vi "Timeout Timer.vi"(2 "timeout(s)":dbl=5.0) -> (7 "timeout?":bool, 9 "time esliped?":dbl)   [LabVIEW 2017]
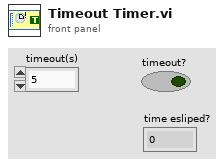
[diagram p1: front panel]
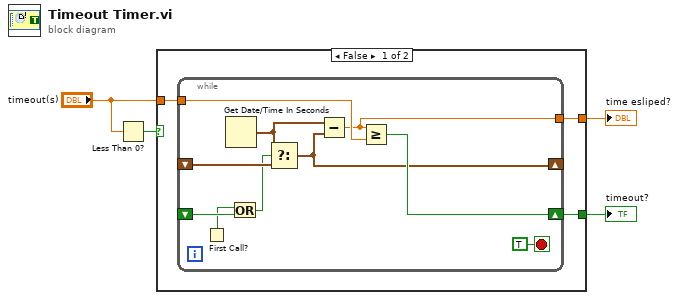
[diagram p0: block diagram]
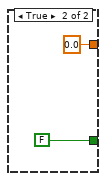
[diagram p2: hidden frame]
diagram:
  n1 = Less Than 0?(x="timeout(s)") -> (x < 0?=w3:bool)
  n2 = case shown="False" w3 {
    tunnel: "timeout(s)" -> [w7 _]
    tunnel: [w6 FALSE] -> w4
    tunnel: [w5 0.0] -> w1
    frame False {
      n3 = while {
        shift-right: [w8] -> _
        shift-left: _ -> [w16]
        tunnel: w7 -> [w15]
        shift-right: [w14] -> w6
        shift-left: _ -> [w13]
        tunnel: [w10] -> w5
        stop <- TRUE stop-if-true
        n4 = First Call?() -> (First Call?: T/F=w12:bool)
        n5 = Get Date/Time In Seconds() -> (seconds since 1Jan1904=w9:timestamp)
        n6 = Or(x=w12, y=w13) -> (x .or. y?=w11:bool)
        n7 = Select(t=w9, s=w11, f=w16) -> (s? t:f=w8:timestamp)
        n8 = Subtract(x=w9, y=w8) -> (x-y=w10:dbl)
        n9 = Greater Or Equal?(x=w10, y=w15) -> (x >= y?=w14:bool)
      }
    }
    frame True {
    }
  }
  "timeout?" <- w4
  "time esliped?" <- w1
